vi "Configure Power Line Frequency.vi"(8 "error in (no error)":errorcluster, 10 "Power Line Frequency  (60 Hz)":u16(ring)=60 items=["60 Hz"=60, "50 Hz or 400 Hz"=50], 11 "VISA resource name":refnum<visa-resource-name>) -> (0 "error out":errorcluster, 3 "VISA resource name out":refnum<visa-resource-name>)   [LabVIEW 2025, in "Keithley 24XX.lvlib"]
doc: "Configures the instrument to the correct power line frequency."
uses:
  Keithley 24XX.lvlib
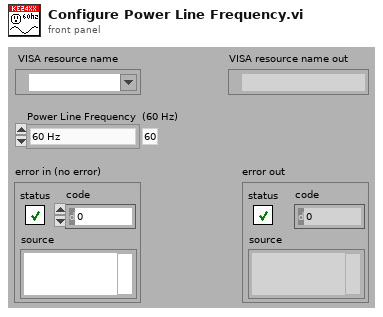
[diagram p1: front panel]
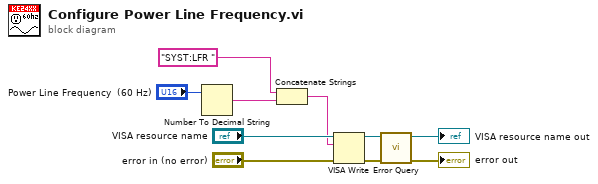
[diagram p0: block diagram]
diagram:
  n1 = Number To Decimal String(number="Power Line Frequency  (60 Hz)") -> (decimal integer string=w2:string)  [unwired: 1 in]
  n2 = Concatenate Strings("SYST:LFR ", w2) -> (w1:string)
  n3 = VISA Write(VISA resource name="VISA resource name", write buffer=w1, error in (no error)="error in (no error)") -> (VISA resource name out=w6:refnum<visa-resource-name>, error out=w5:errorcluster)  [unwired: 1 out]
  n4 = call "Error Query.vi"("error in (no error)"=w5, "VISA resource name"=w6) -> ("error out"=→"error out":errorcluster, "VISA resource name out"=→"VISA resource name out":refnum<visa-resource-name>)  [unwired: 6 in, 2 out]
